vi "Add Items.vi"(8 "error in (no error)":errorcluster, 9 "Array":refnum<k24>[](array[refnum]), 10 "CreateSubscription in":refnum<k24>, 11 ".NET Refnum in":refnum<k24>) -> (0 "error out":errorcluster, 1 "AddItems":refnum<k24>[](array[refnum]), 2 "CreateSubscription out":refnum<k24>, 3 ".NET Refnum out":refnum<k24>)   [LabVIEW 2024, in "LV_OPC_NET.lvlib"]
uses:
  LV_OPC_NET.lvlib
  C:/Users/Andrey/Desktop/LV_OPC-Client-x64/LV_OPC_Test/OPC.NET/OpcNetApi.dll
  OpcNetApi.dll
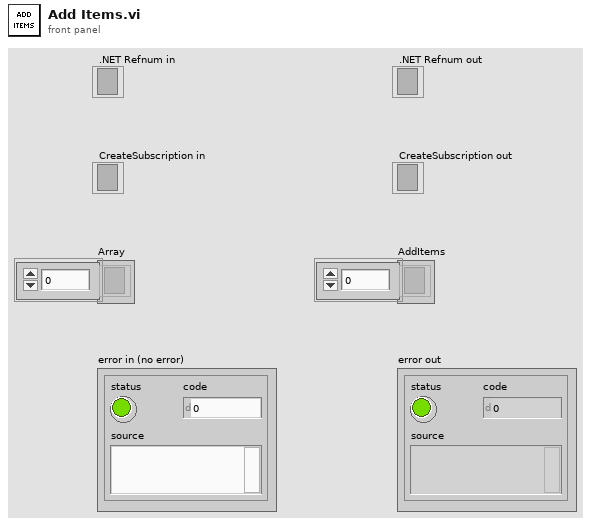
[diagram p1: front panel]
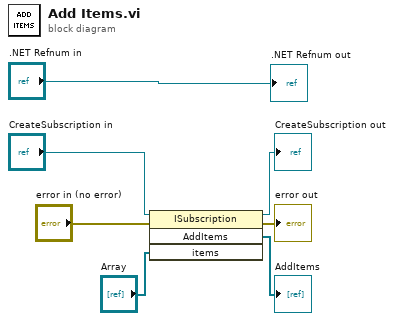
[diagram p0: block diagram]
diagram:
  n1 = invoke class="ISubscription" method="AddItems"(reference="CreateSubscription in", error in="error in (no error)", "items"="Array") -> (reference out=→"CreateSubscription out":refnum<k24>, error out=→"error out":errorcluster, "AddItems"=→"AddItems":refnum<k24>[])  [unwired: 1 in, 1 out]
  ".NET Refnum out" <- ".NET Refnum in"
